vi "제목없음 1.vi"() -> ()   [LabVIEW 2017]
uses:
  <vilib>/DAQmx/write.llb/DAQmx Write (Analog Wfm 1Chan NSamp).vi
  <vilib>/DAQmx/create/channels.llb/DAQmx Create Channel (AO-Voltage-Basic).vi
  <vilib>/DAQmx/configure/timing.llb/DAQmx Timing (Sample Clock).vi
  <vilib>/DAQmx/miscellaneous.llb/DAQmx Fill In Error Info.vi
  <vilib>/Analysis/NI_AALBase.lvlib
panel:
  in  "정지 버튼":bool
  out "TX Signal 2":waveform(dbl)(graph)
  in  "fs":dbl=0.0004 format="%#_6p"
  in  "송신 채널 설정":tag="Dev3/ao0"
  in  "송신 디바이스 이름":tag="Dev3"
  in  "Pulse length(sec)":dbl=0.0004 format="%#_6p"
  in  "Stop Frequency(Hz)":dbl=470000.0 format="%#_6p"
  in  "Start Frequency(Hz)":dbl=430000.0 format="%#_6p"
  out "TX Signal":waveform(dbl)(graph)
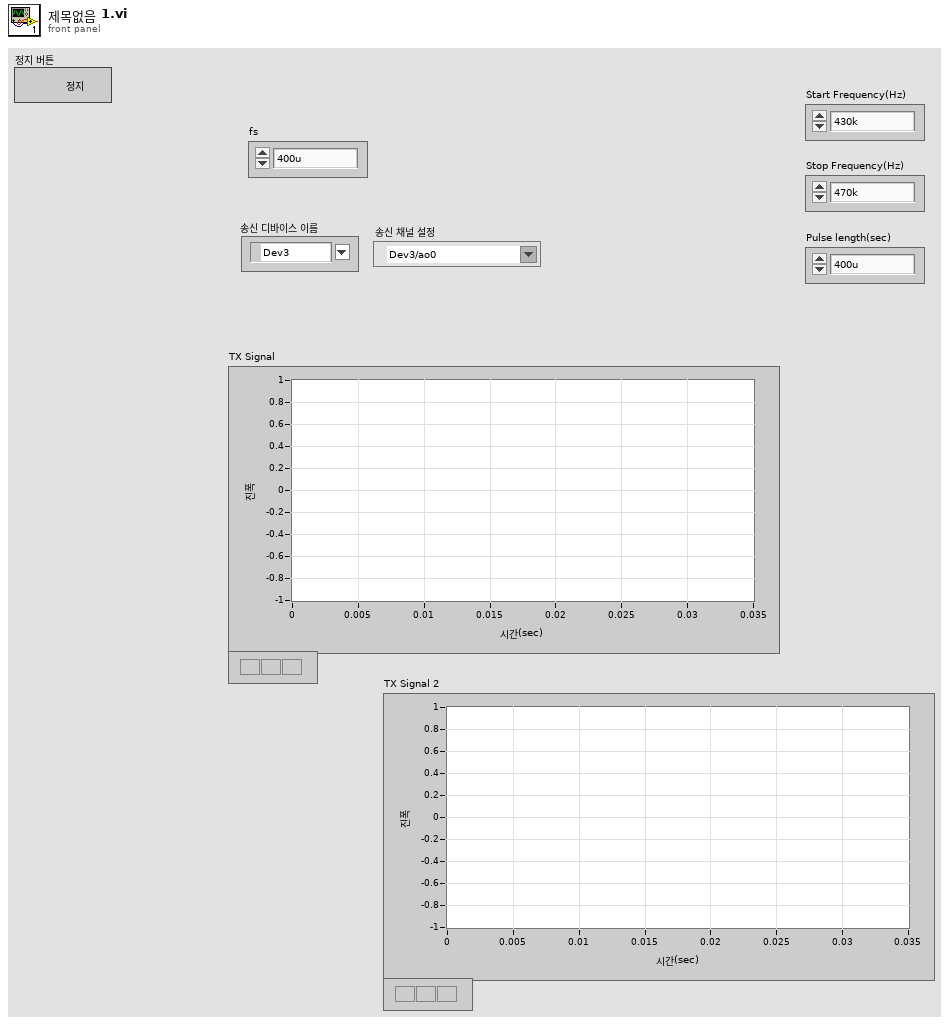
[diagram p1: front panel]
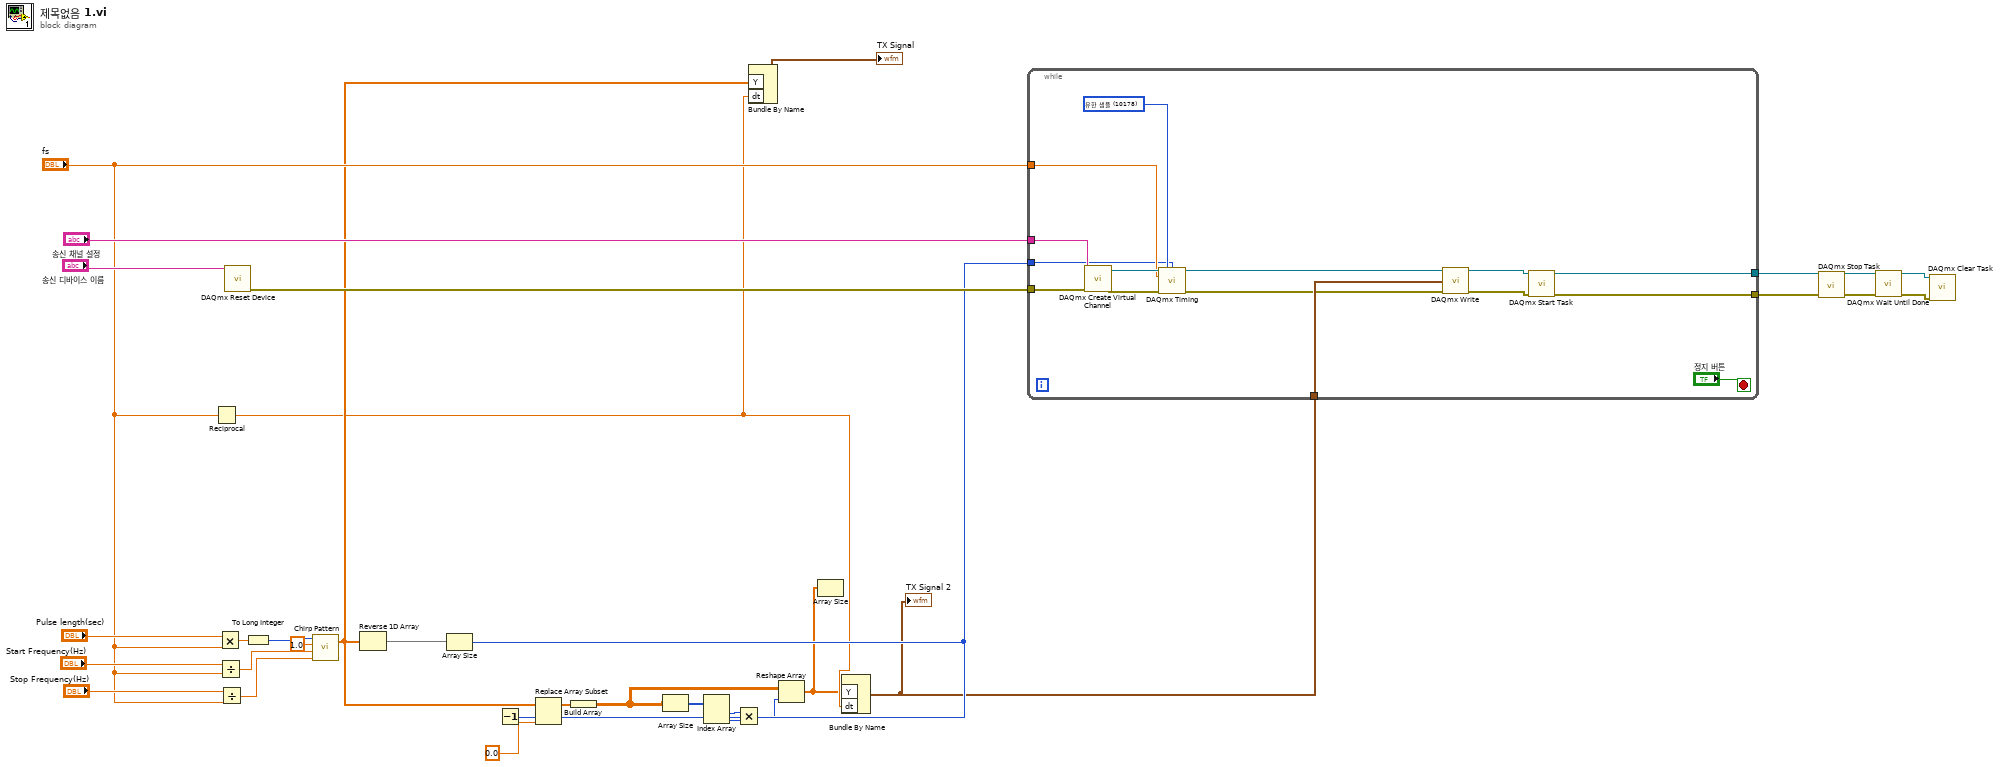
[diagram p0: block diagram]
diagram:
  n1 = Reciprocal(x="fs") -> (1/x=w9:dbl)
  n2 = Multiply(x="Pulse length(sec)", y="fs") -> (x*y=w32:dbl)
  n3 = Divide(x="Start Frequency(Hz)", y="fs") -> (x/y=w22:dbl)
  n4 = Divide(x="Stop Frequency(Hz)", y="fs") -> (x/y=w27:dbl)
  n5 = call <vilib>:"DAQmx Reset Device.vi"("device in"="송신 디바이스 이름") -> ("error out"=w26:errorcluster)  [unwired: 1 in, 13 out]
  n6 = To Long Integer(number=w32) -> (32bit integer=w31:i32)
  n7 = call <vilib>:"Chirp Pattern.vi"("f2"=w27, "f1"=w22, "amplitude"=1.0, "samples"=w31) -> ("Chirp Pattern"=w19:dbl[])  [unwired: 1 out]
  n8 = Reverse 1D Array(array=w19) -> (reversed array=w23:dbl[])
  n9 = Array Size(array=w23) -> (size(s)=w18:i32)
  n10 = Decrement(x=w18) -> (x-1=w17:i32)
  n11 = Replace Array Subset(array=w19, new element=0.0 ("새 원소/부분배열"), index=w17) -> (w15:dbl[])
  n12 = Build Array(w15) -> (w10:dbl[][])
  n13 = Array Size(array=w10) -> (size(s)=w11:i32[])
  n14 = Index Array(array=w11) -> (element #1=w13:i32, element #2=w12:i32)  [unwired: 2 in]
  n15 = Multiply(x=w13, y=w12) -> (x*y=w14:i32)
  n16 = Bundle By Name("Y"=w19, "dt"=w9) -> (→"TX Signal":waveform(dbl))  [unwired: 1 in]
  n17 = Reshape Array(w10, w14) -> (w7:dbl[])
  n18 = Array Size(array=w7) -> ()  [unwired: 1 out]
  n19 = Bundle By Name("Y"=w7, "dt"=w9) -> (w8:waveform(dbl))  [unwired: 1 in]
  "TX Signal 2" <- w8
  n20 = while {
    tunnel: w26 -> [w48]
    tunnel: "송신 채널 설정" -> [w45]
    tunnel: "fs" -> [w41]
    tunnel: w18 -> [w36]
    tunnel: w8 -> [w40]
    tunnel: [w35] -> w2
    tunnel: [w34] -> w1
    stop <- "정지 버튼" stop-if-true
    w42 = 10178 items=["유한 샘플"=10178, "연속 샘플"=10123, "하드웨어 타이밍에 의한 단일 포인트"=12522] ("sample mode")
    n21 = call-poly <vilib>:"DAQmx Create Virtual Channel.vi"("physical channels"=w45, "error in"=w48) -> ("task out"=w46:refnum<k21>, "error out"=w47:errorcluster)  [unwired: 7 in, 5 out]
    n22 = call-poly <vilib>:"DAQmx Timing.vi"("task/channels in"=w46, "sample mode"=w42, "samples per channel"=w36, "rate"=w41, "error in"=w47) -> ("task out"=w38:refnum<k21>, "error out"=w37:errorcluster)  [unwired: 2 in, 7 out]
    n23 = call-poly <vilib>:"DAQmx Write.vi"("task/channels in"=w38, "data"=w40, "error in"=w37) -> ("task out"=w44:refnum<k21>, "error out"=w43:errorcluster)  [unwired: 10 in, 1 out]
    n24 = call <vilib>:"DAQmx Start Task.vi"("task/channels in"=w44, "error in"=w43) -> ("task out"=w35:refnum<k21>, "error out"=w34:errorcluster)  [unwired: 12 in]
  }
  n25 = call <vilib>:"DAQmx Stop Task.vi"("task/channels in"=w2, "error in"=w1) -> ("task out"=w3:refnum<k21>, "error out"=w4:errorcluster)  [unwired: 12 in]
  n26 = call <vilib>:"DAQmx Wait Until Done.vi"("task/channels in"=w3, "error in"=w4) -> ("task out"=w5:refnum<k21>, "error out"=w6:errorcluster)  [unwired: 12 in]
  n27 = call <vilib>:"DAQmx Clear Task.vi"("task in"=w5, "error in"=w6) -> ()  [unwired: 13 in, 1 out]
